vi "RoomJSONTest.vi"() -> (0 "error out":errorcluster, 2 "Pass":bool)   [LabVIEW 2015]
uses:
  Flags/ColorEnum.ctl
  NurseStation/TypeDef/SelectedRoom.ctl
  Flags/ColorFlags.ctl
  Room/Room.lvclass/Room.ctl
  Room/Write Beacon Id.vi
  Room/Write BedVacant.vi
  Room/Write InRoomPersonnel.vi
  Room/Write RoomRequests.vi
  Room/Read Beacon Id.vi
  Room/Read BedVacant.vi
  Room/Read InRoomPersonnel.vi
  Room/Read Room Number.vi
  Room/Read RoomRequests.vi
  Room/Read Flags.lvclass.vi
  Flags/Flags.lvclass
  Room/Room.lvclass
panel:
  out "error out 2":errorcluster
  out "After Json 2":T1={"Room Number"=0, "RoomNumFlags"={"Flag State"=[1, 3, 5, 7]}, "BedVacant"=FALSE, "InRoomPersonnel"=[], "RoomRequests"=[]}
  out "String":string
  in  "RoomRequests":string[](array[string])=["Cleanning"]
  in  "InRoomPersonnel":string[](array[string])=["Dr Y"]
  in  "BedVacant":bool
  in  "Beacon Id":string="test"
  out "After Json":T1={"Room Number"=0, "RoomNumFlags"={"Flag State"=[1, 3, 5, 7]}, "BedVacant"=FALSE, "InRoomPersonnel"=[], "RoomRequests"=[]}
  out "Before Json":T1={"Room Number"=0, "RoomNumFlags"={"Flag State"=[1, 3, 5, 7]}, "BedVacant"=FALSE, "InRoomPersonnel"=[], "RoomRequests"=[]}
  in  "Color":T3[](array[typedef])=[enum."Red", enum."Blue", enum."Green", enum."Yellow"]
  in  "State":bool[](array[boolean])=[FALSE, FALSE, FALSE, TRUE]
  in  "Room Number":u8=1
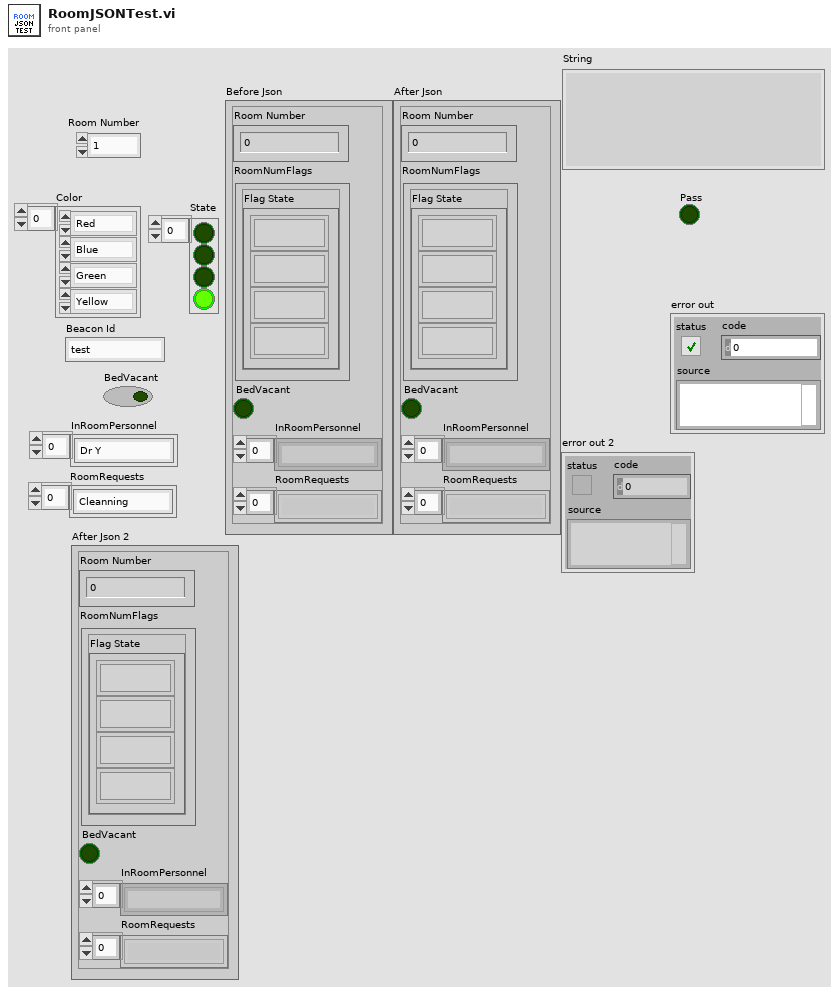
[diagram p1: front panel]
types:
  T1 = typedef "Room.lvclass/SelectedRoom.ctl" = cluster{"Room Number":u8, "RoomNumFlags":T2, "BedVacant":bool, "InRoomPersonnel":string[], "RoomRequests":string[]}
  T2 = typedef "Flags.lvclass/ColorFlags.ctl" = cluster{"Flag State":u8[]}
  T3 = typedef "Flags.lvclass/ColorEnum.ctl" = enum8{"Red", "Blue", "Green", "Yellow"}
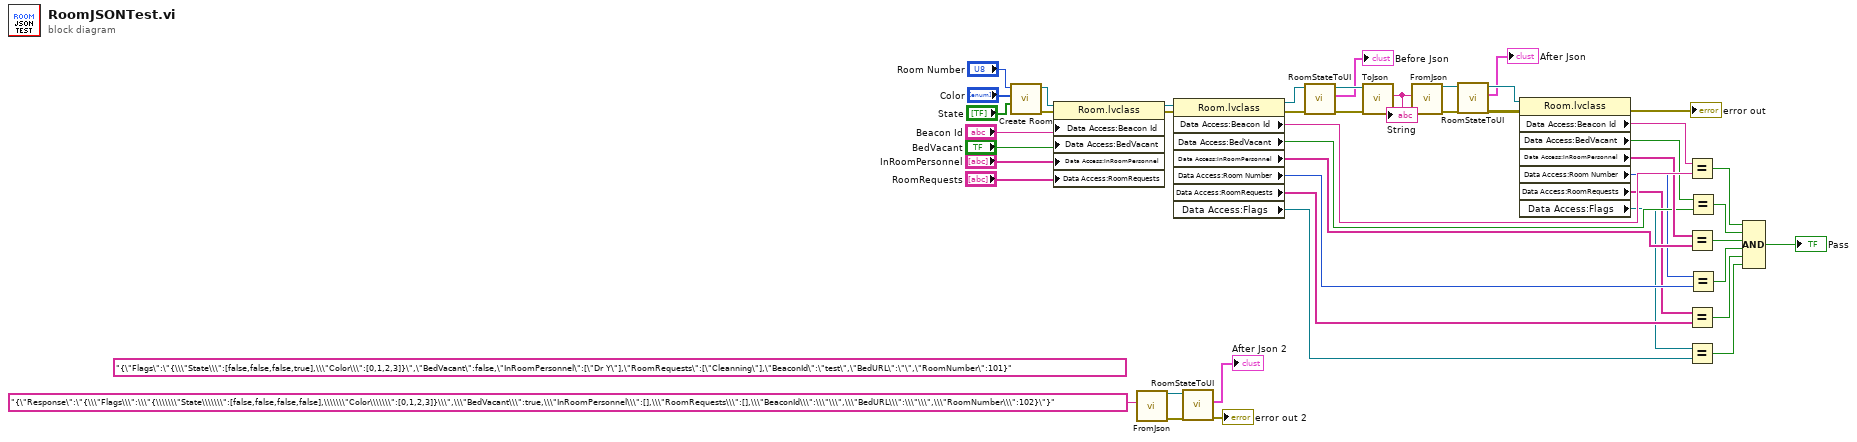
[diagram p0: block diagram]
diagram:
  (unwired) "{\"Flags\":\"{\\\"State\\\":[false,false,false,true],\\\"Color\\\":[0,1,2,3]}\",\"BedVacant\":false,\"InRoomPersonnel\":[\"Dr Y\"],\"RoomRequests\":[\"Cleanning\"],\"BeaconId\":\"test\",\"BedURL\":\"\",\"RoomNumber\":101}" ("String")
  n1 = call "Create Room.vi"("State"="State", "Color"="Color", "Room Number"="Room Number") -> ("error out"=w12:errorcluster, "Room Ref"=w13:refnum<class "Room.lvclass">)  [unwired: 7 in]
  n2 = property class="Room.lvclass"(reference=w13, error in=w12, "Data Access:Beacon Id"="Beacon Id", "Data Access:BedVacant"="BedVacant", "Data Access:InRoomPersonnel"="InRoomPersonnel", "Data Access:RoomRequests"="RoomRequests") -> (reference out=w11:refnum<class "Room.lvclass">, error out=w10:errorcluster)
  n3 = call "FromJson.vi"("String"="{\"Response\":\"{\\\"Flags\\\":\\\"{\\\\\\\"State\\\\\\\":[false,false,false,false],\\\\\\\"Color\\\\\\\":[0,1,2,3]}\\\",\\\"BedVacant\\\":true,\\\"InRoomPersonnel\\\":[],\\\"RoomRequests\\\":[],\\\"BeaconId\\\":\\\"\\\",\\\"BedURL\\\":\\\"\\\",\\\"RoomNumber\\\":102}\"}") -> ("error out"=w2:errorcluster, "Room out"=w5:refnum<class "Room.lvclass">)  [unwired: 9 in]
  n4 = property class="Room.lvclass"(reference=w11, error in=w10) -> (reference out=w23:refnum<class "Room.lvclass">, error out=w22:errorcluster, "Data Access:Beacon Id"=w47:string, "Data Access:BedVacant"=w41:bool, "Data Access:InRoomPersonnel"=w40:string[], "Data Access:Room Number"=w32:i32, "Data Access:RoomRequests"=w30:string[], "Data Access:Flags"=w26:refnum<class "Flags.lvclass">)
  n5 = call "RoomStateToUI.vi"("error in"=w2, "Room In"=w5) -> ("error out"=→"error out 2":errorcluster, "Selected Room"=→"After Json 2":T1)  [unwired: 7 in, 1 out]
  n6 = call "RoomStateToUI.vi"("error in"=w22, "Room In"=w23) -> ("error out"=w21:errorcluster, "Selected Room"=→"Before Json":T1, "Room Out"=w20:refnum<class "Room.lvclass">)  [unwired: 7 in]
  n7 = call "ToJson.vi"("error in (no error)"=w21, "Room in"=w20) -> ("error out"=w34:errorcluster, "String"=w24:string)  [unwired: 7 in, 1 out]
  "String" <- w24
  n8 = call "FromJson.vi"("error in (no error)"=w34, "String"=w24) -> ("error out"=w19:errorcluster, "Room out"=w16:refnum<class "Room.lvclass">)  [unwired: 8 in]
  n9 = call "RoomStateToUI.vi"("error in"=w19, "Room In"=w16) -> ("error out"=w18:errorcluster, "Selected Room"=→"After Json":T1, "Room Out"=w17:refnum<class "Room.lvclass">)  [unwired: 7 in]
  n10 = property class="Room.lvclass"(reference=w17, error in=w18) -> (error out=→"error out":errorcluster, "Data Access:Beacon Id"=w48:string, "Data Access:BedVacant"=w46:bool, "Data Access:InRoomPersonnel"=w42:string[], "Data Access:Room Number"=w33:i32, "Data Access:RoomRequests"=w31:string[], "Data Access:Flags"=w25:refnum<class "Flags.lvclass">)  [unwired: 1 out]
  n11 = Equal?(x=w48, y=w47) -> (x = y?=w45:bool)
  n12 = Equal?(x=w42, y=w40) -> (x = y?=w38:bool)
  n13 = Equal?(x=w31, y=w30) -> (x = y?=w28:bool)
  n14 = Equal?(x=w25, y=w26) -> (x = y?=w27:bool)
  n15 = Equal?(x=w46, y=w41) -> (x = y?=w39:bool)
  n16 = Equal?(x=w33, y=w32) -> (x = y?=w29:bool)
  n17 = Compound Arithmetic op=AND(w45, w39, w38, w29, w28, w27) -> (→"Pass":bool)
